vi "Eval y=f(x) Prep2 (VI).vi"(0 "points in":dbl[](array[numeric]), 1 "f(x)":T1, 2 "random summand":dbl format="%.2f", 5 "points I in":dbl[](array[numeric]), 7 "points II in":dbl[](array[numeric]), 11 "error in":i32, 12 "data":variant, 13 "epsilon":dbl format="%.2f", 14 "sign":i32(ring) items=["y=f(x)", "y=-f(x)"]) -> (4 "points out":dbl[](array[numeric]), 6 "points I out":dbl[](array[numeric]), 15 "error out":i32)   [LabVIEW 2020, in "NI_Gmath.lvlib"]
uses:
  NI_Gmath.lvlib
  functionRefnum.ctl
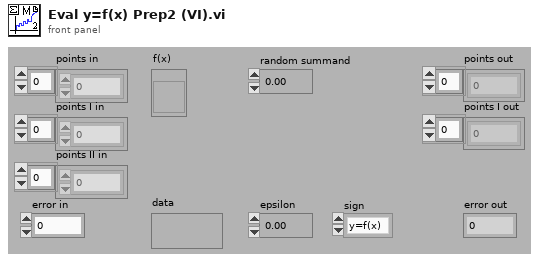
[diagram p1: front panel]
types:
  T1 = typedef "NI_Gmath.lvlib/functionRefnum.ctl" = refnum<vi>
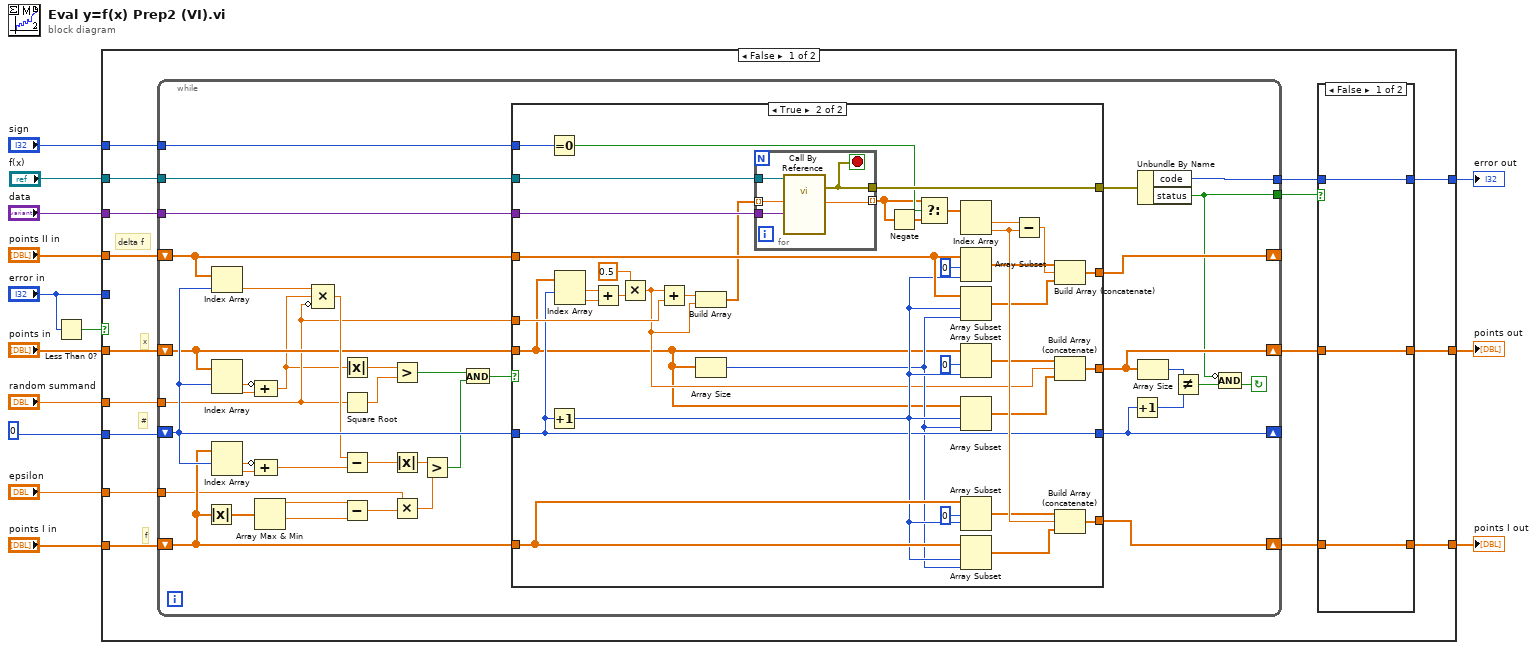
[diagram p0: block diagram]
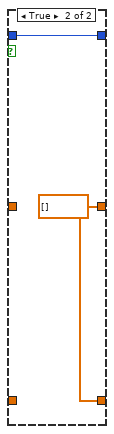
[diagram p2: hidden frame]
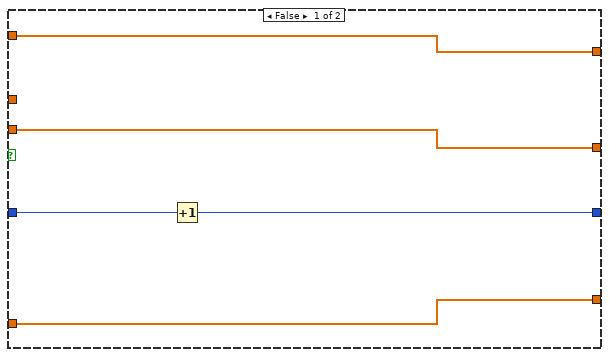
[diagram p3: hidden frame]
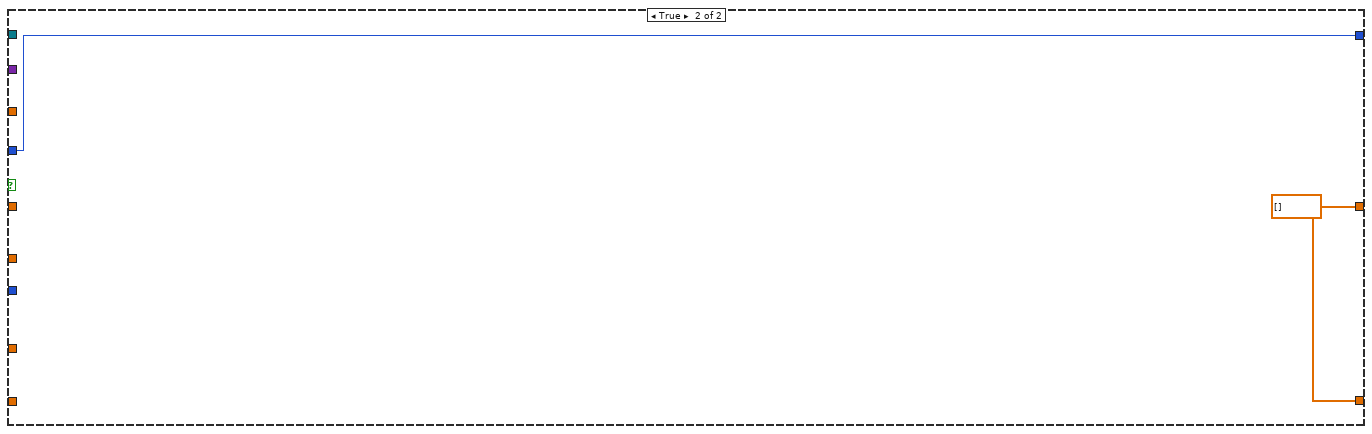
[diagram p4: hidden frame]
diagram:
  n1 = Less Than 0?(x="error in") -> (x < 0?=w10:bool)
  n2 = case shown="False" w10 {
    tunnel: "epsilon" -> [w30 _]
    tunnel: [w20 w123] -> w1
    tunnel: [w18 w123] -> w2
    tunnel: "points I in" -> [w29 _]
    tunnel: 0 -> [w28 _]
    tunnel: "points II in" -> [w27 _]
    tunnel: "points in" -> [w26 _]
    tunnel: "random summand" -> [w25 _]
    tunnel: "f(x)" -> [w24 _]
    tunnel: "data" -> [w23 _]
    tunnel: "error in" -> [_ w124]
    tunnel: [w16 w124] -> w3
    tunnel: "sign" -> [w22 _]
    frame False {
      # "#"
      # "delta f"
      # "f"
      # "x"
      n3 = while {
        tunnel: w30 -> [w44]
        tunnel: w25 -> [w45]
        shift-left: w28 -> [w69]
        shift-right: [w71] -> _
        shift-left: w27 -> [w72]
        shift-right: [w74] -> _
        shift-left: w29 -> [w50]
        shift-right: [w75] -> w21
        shift-left: w26 -> [w51]
        shift-right: [w73] -> w19
        tunnel: w24 -> [w49]
        tunnel: w23 -> [w48]
        tunnel: w22 -> [w41]
        tunnel: [w38] -> w17
        tunnel: [w37] -> w15
        stop <- w39 continue-if-true
        n4 = Absolute Value(x=w50) -> (abs(x)=w65:dbl[])
        n5 = Index Array(array=w72, index=w69) -> (element=w43:dbl)
        n6 = Index Array(array=w51, index #1=w69) -> (element #1=w62:dbl, element #2=w47:dbl)  [unwired: 1 in]
        n7 = Index Array(array=w50, index #1=w69) -> (element #1=w61:dbl, element #2=w46:dbl)  [unwired: 1 in]
        n8 = Compound Arithmetic op=ADD(invert w62, w47) -> (w42:dbl)
        n9 = Compound Arithmetic op=ADD(invert w61, w46) -> (w67:dbl)
        n10 = Array Max & Min(array=w65) -> (max value=w60:dbl, min value=w59:dbl)  [unwired: 2 out]
        n11 = Compound Arithmetic op=MULTIPLY(w43, w42, invert w45) -> (w68:dbl)
        n12 = Absolute Value(x=w42) -> (abs(x)=w55:dbl)
        n13 = Square Root(x=w45) -> (sqrt(x)=w52:dbl)
        n14 = Subtract(x=w68, y=w67) -> (x-y=w66:dbl)
        n15 = Subtract(x=w60, y=w59) -> (x-y=w58:dbl)
        n16 = Greater?(x=w55, y=w52) -> (0:w54:bool)
        n17 = Absolute Value(x=w66) -> (abs(x)=w64:dbl)
        n18 = Multiply(x=w44, y=w58) -> (x*y=w63:dbl)
        n19 = Greater?(x=w64, y=w63) -> (0:w56:bool)
        n20 = And(x=w54, y=w56) -> (x .and. y?=w53:bool)
        n21 = case shown="True" w53 {
          tunnel: w69 -> [w77 w96]
          tunnel: w51 -> [w80 w81]
          tunnel: [w80 w109] -> w73
          tunnel: w50 -> [w79 w106]
          tunnel: [w79 w99] -> w75
          tunnel: w72 -> [w78 w102]
          tunnel: [w78 w98] -> w74
          tunnel: w45 -> [_ w103]
          tunnel: [w76 w96] -> w71
          tunnel: w49 -> [_ w116]
          tunnel: w48 -> [_ w115]
          tunnel: w41 -> [_ w87]
          tunnel: [_ w86] -> w36
          frame False {
            n22 = Increment(x=w77) -> (x+1=w76:i32)
          }
          frame True {
            n23 = Equal To 0?(x=w87) -> (x = 0?=w84:bool)
            n24 = Increment(x=w96) -> (x+1=w97:i32)
            n25 = Index Array(array=w81, index #1=w96) -> (element #1=w114:dbl, element #2=w93:dbl)  [unwired: 1 in]
            n26 = Add(x=w114, y=w93) -> (x+y=w113:dbl)
            n27 = Multiply(x=0.5, y=w113) -> (x*y=w89:dbl)
            n28 = Add(x=w89, y=w103) -> (x+y=w91:dbl)
            n29 = Build Array(w91, w89) -> (w95:dbl[])
            n30 = Array Size(array=w81) -> (size(s)=w92:i32)
            n31 = for {
              tunnel: w116 -> [w122]
              tunnel: w115 -> [w120]
              tunnel: w95 -> [w121] mode=indexing
              tunnel: [w119] -> w86
              tunnel: [w118] -> w82 mode=indexing
              stop <- w119 stop-if-true
              n32 = call-by-ref "?"(reference=w122, "Variant"=w120, "x"=w121) -> (error out=w119:errorcluster, "f(x)"=w118:dbl)  [unwired: 4 in, 1 out]
            }
            n33 = Negate(x=w82) -> (-x=w85:dbl[])
            n34 = Select(t=w82, s=w84, f=w85) -> (s? t:f=w83:dbl[])
            n35 = Index Array(array=w83) -> (element #1=w94:dbl, element #2=w117:dbl)  [unwired: 2 in]
            n36 = Array Subset(array=w102, index=0, length=w97) -> (w100:dbl[])
            n37 = Array Subset(array=w102, index=w97, length=w92) -> (w88:dbl[])
            n38 = Array Subset(array=w81, index=0, length=w97) -> (w111:dbl[])
            n39 = Array Subset(array=w81, index=w97, length=w92) -> (w110:dbl[])
            n40 = Array Subset(array=w106, index=0, length=w97) -> (w105:dbl[])
            n41 = Array Subset(array=w106, index=w97, length=w92) -> (w104:dbl[])
            n42 = Subtract(x=w94, y=w117) -> (x-y=w90:dbl)
            n43 = Build Array (concatenate)(w100, w90, w88) -> (w98:dbl[])
            n44 = Build Array (concatenate)(w111, w89, w110) -> (w109:dbl[])
            n45 = Build Array (concatenate)(w105, w117, w104) -> (w99:dbl[])
          }
        }
        n46 = Increment(x=w71) -> (x+1=w70:i32)
        n47 = Unbundle By Name(w36) -> ("code"=w38:i32, "status"=w37:bool)
        n48 = Array Size(array=w73) -> (size(s)=w57:i32)
        n49 = Not Equal?(x=w57, y=w70) -> (x != y?=w40:bool)
        n50 = Compound Arithmetic op=AND(invert w37, w40) -> (w39:bool)
      }
      n51 = case shown="False" w15 {
        tunnel: w21 -> [w33 _]
        tunnel: [w33 w34] -> w20
        tunnel: [w31 w34] -> w18
        tunnel: w17 -> [w32 w35]
        tunnel: [w32 w35] -> w16
        tunnel: w19 -> [w31 _]
        frame False {
        }
        frame True {
          w34 = dbl[] [] ("points in")
        }
      }
    }
    frame True {
      w123 = dbl[] [] ("points in")
    }
  }
  "error out" <- w3
  "points out" <- w2
  "points I out" <- w1
